vi "TIRF-Lock.vi"(8 "error in (no error)":errorcluster, 11 "Config":T1 {"Hardware Configuration"."Lasers Configuration"."SettingValues"."785 Power" format="%.1f"; "Hardware Configuration"."Lasers Configuration"."SettingValues"."647 Power" format="%.1f"; "Hardware Configuration"."Lasers Configuration"."SettingValues"."561 Power" format="%.1f"; "Hardware Configuration"."Lasers Configuration"."SettingValues"."532 Power" format="%.1f"; "Hardware Configuration"."Lasers Configuration"."SettingValues"."488 Power" format="%.1f"; "Hardware Configuration"."Lasers Configuration"."SettingValues"."405 Power" format="%.1f"}) -> (0 "error Out":errorcluster, 3 "Config 2":T1 {"Hardware Configuration"."Lasers Configuration"."SettingValues"."785 Power" format="%.1f"; "Hardware Configuration"."Lasers Configuration"."SettingValues"."647 Power" format="%.1f"; "Hardware Configuration"."Lasers Configuration"."SettingValues"."561 Power" format="%.1f"; "Hardware Configuration"."Lasers Configuration"."SettingValues"."532 Power" format="%.1f"; "Hardware Configuration"."Lasers Configuration"."SettingValues"."488 Power" format="%.1f"; "Hardware Configuration"."Lasers Configuration"."SettingValues"."405 Power" format="%.1f"})   [LabVIEW 2019]
uses:
  Settings/Settings.ctl
  HardwareAdapter/Support/Hardware Configuration.ctl
  HardwareAdapter/Support/Camera Configuration.ctl
  D:/SDK/PMQI-LabViewSamples/Examples/Dependencies/PVCamNET.dll
  <vilib>/vision/Image Controls.llb/IMAQ Image.ctl
  <vilib>/userdefined/High Color/IMAQdx.ctl
  E:/DevHardSoftware/MMicroscopy/HardwareAdapter/Lasers/Dependencies/Oxxius_Boxx.dll
  HardwareAdapter/Lasers/Dependencies/Oxxius_Boxx.dll
  Logging/Logging Configuration.ctl
  controls/UI Configuration.ctl
  controls/CallBack Refs.ctl
  Global.vi
  Logging/Logging.lvlib
  Settings/Settings.lvlib
panel:
  in  "Sum":dbl=0.01
  out "Lock Point Y":dbl step=0.01 format="%#.4g"
  out "Lock Point X":dbl step=0.01 format="%#.4g"
  out "cal":dbl format="%#.4g"
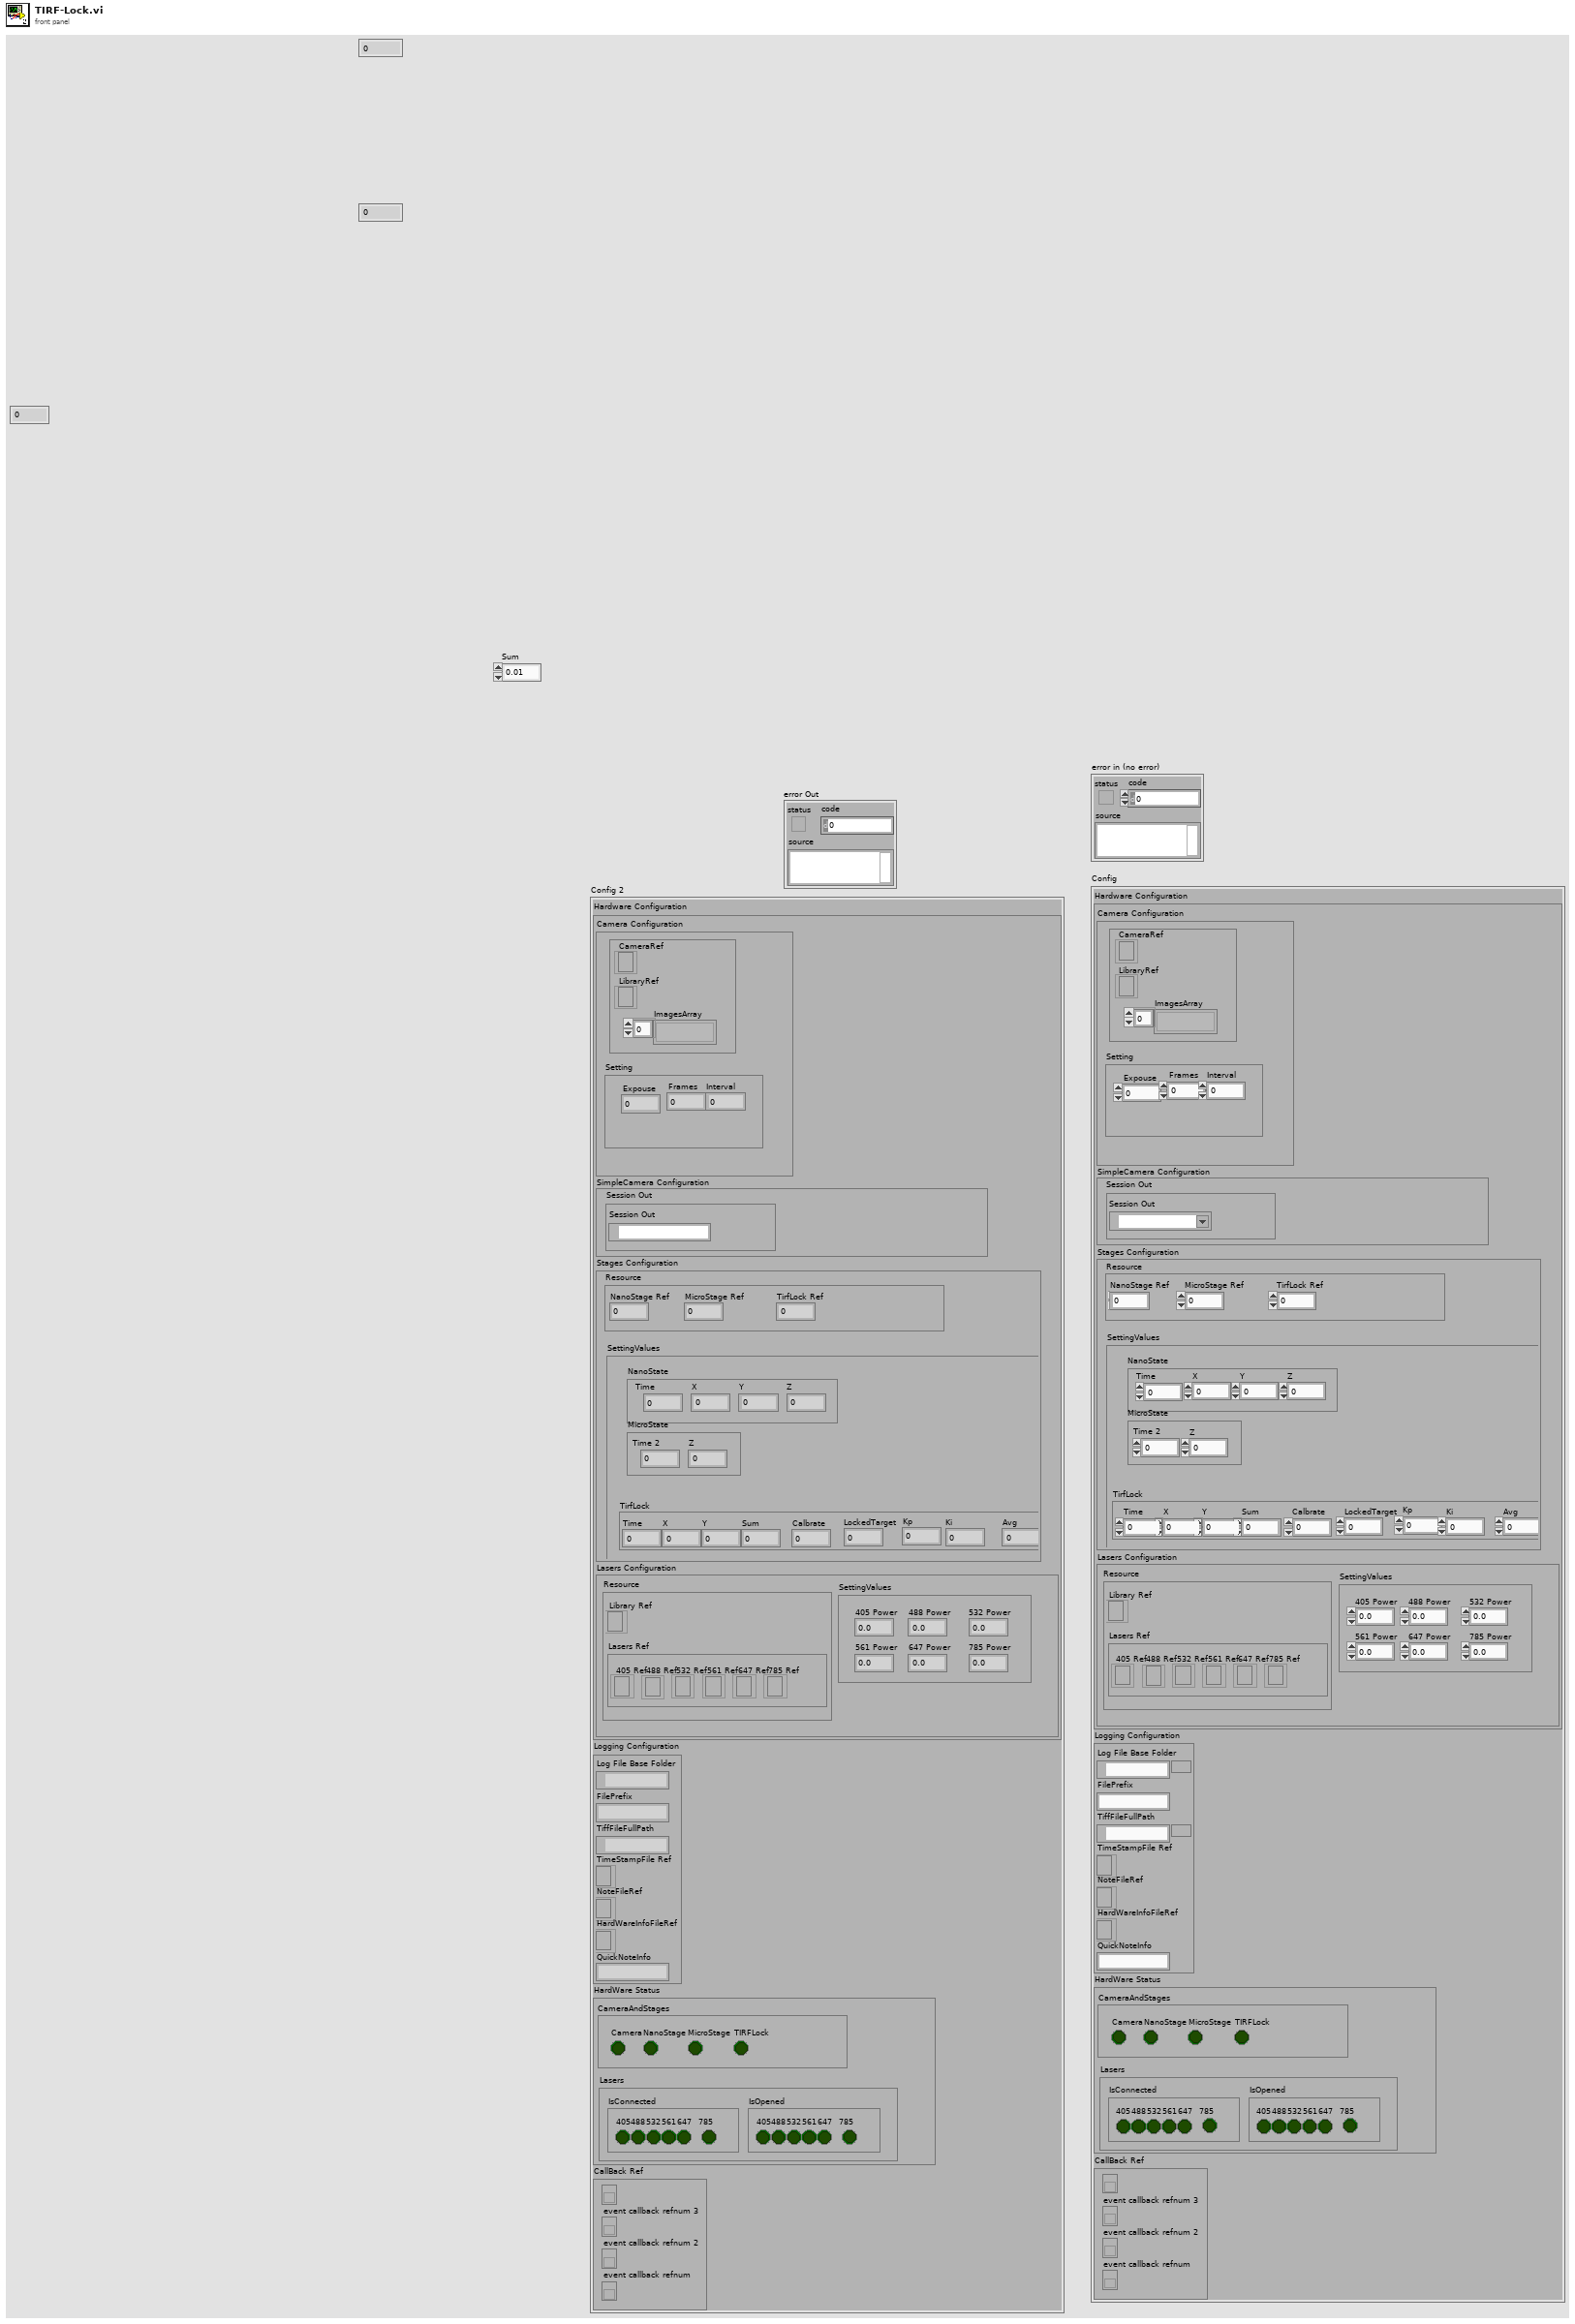
[diagram p1: front panel]
types:
  T1 = typedef "Settings.lvlib/Settings.ctl" = cluster{"Hardware Configuration":T2, "Logging Configuration":T6, "HardWare Status":cluster{"CameraAndStages":T7, "Lasers":cluster{"IsConnected":cluster{"405":bool, "488":bool, "532":bool, "561":bool, "647":bool, "785":bool}, "IsOpened":cluster{"405":bool, "488":bool, "532":bool, "561":bool, "647":bool, "785":bool}}}, "CallBack Ref":T8}
  T2 = typedef "Hardware Configuration.ctl" = cluster{"Camera Configuration":T3, "SimpleCamera Configuration":cluster{"Resource":cluster{"Session Out":T5}}, "Stages Configuration":cluster{"Resource":cluster{"NanoStage Ref":i32, "MicroStage Ref":i32, "TirfLock Ref":i32}, "SettingValues":cluster{"NanoState":cluster{"Time":dbl, "X":dbl, "Y":dbl, "Z":dbl}, "MicroState":cluster{"Time 2":dbl, "Z":dbl}, "TirfLock":cluster{"Time":dbl, "X":dbl, "Y":dbl, "Sum":dbl, "Calbrate":dbl, "LockedTarget":dbl, "Kp":dbl, "Ki":dbl, "Avg":dbl}}}, "Lasers Configuration":cluster{"SettingValues":cluster{"405 Power":sgl, "488 Power":sgl, "532 Power":sgl, "561 Power":sgl, "647 Power":sgl, "785 Power":sgl}, "Resource":cluster{"Library Ref":refnum<k24>, "Lasers Ref":cluster{"405 Ref":refnum<k24>, "488 Ref":refnum<k24>, "532 Ref":refnum<k24>, "561 Ref":refnum<k24>, "647 Ref":refnum<k24>, "785 Ref":refnum<k24>}}}}
  T3 = typedef "Camera Configuration.ctl" = cluster{"Setting":cluster{"Expouse":dbl, "Frames":dbl, "Interval":dbl}, "Resource":cluster{"CameraRef":refnum<k24>, "LibraryRef":refnum<k24>, "ImagesArray":T4[]}}
  T4 = typedef "IMAQ Image.ctl" = refnum<image>
  T5 = typedef "IMAQdx.ctl" = refnum<k21>
  T6 = typedef "Logging.lvlib/Logging Configuration.ctl" = cluster{"Log File Base Folder":path, "FilePrefix":string, "TiffFileFullPath":path, "TimeStampFile Ref":refnum<file>, "NoteFileRef":refnum<file>, "HardWareInfoFileRef":refnum<file>, "QuickNoteInfo":string}
  T7 = typedef "UI Configuration.ctl" = cluster{"Camera":bool, "NanoStage":bool, "MicroStage":bool, "TIRFLock":bool}
  T8 = typedef "CallBack Refs.ctl" = cluster{"event callback refnum":refnum<k27>, "event callback refnum 2":refnum<k27>, "event callback refnum 3":refnum<k27>, "event callback refnum 4":refnum<k27>}
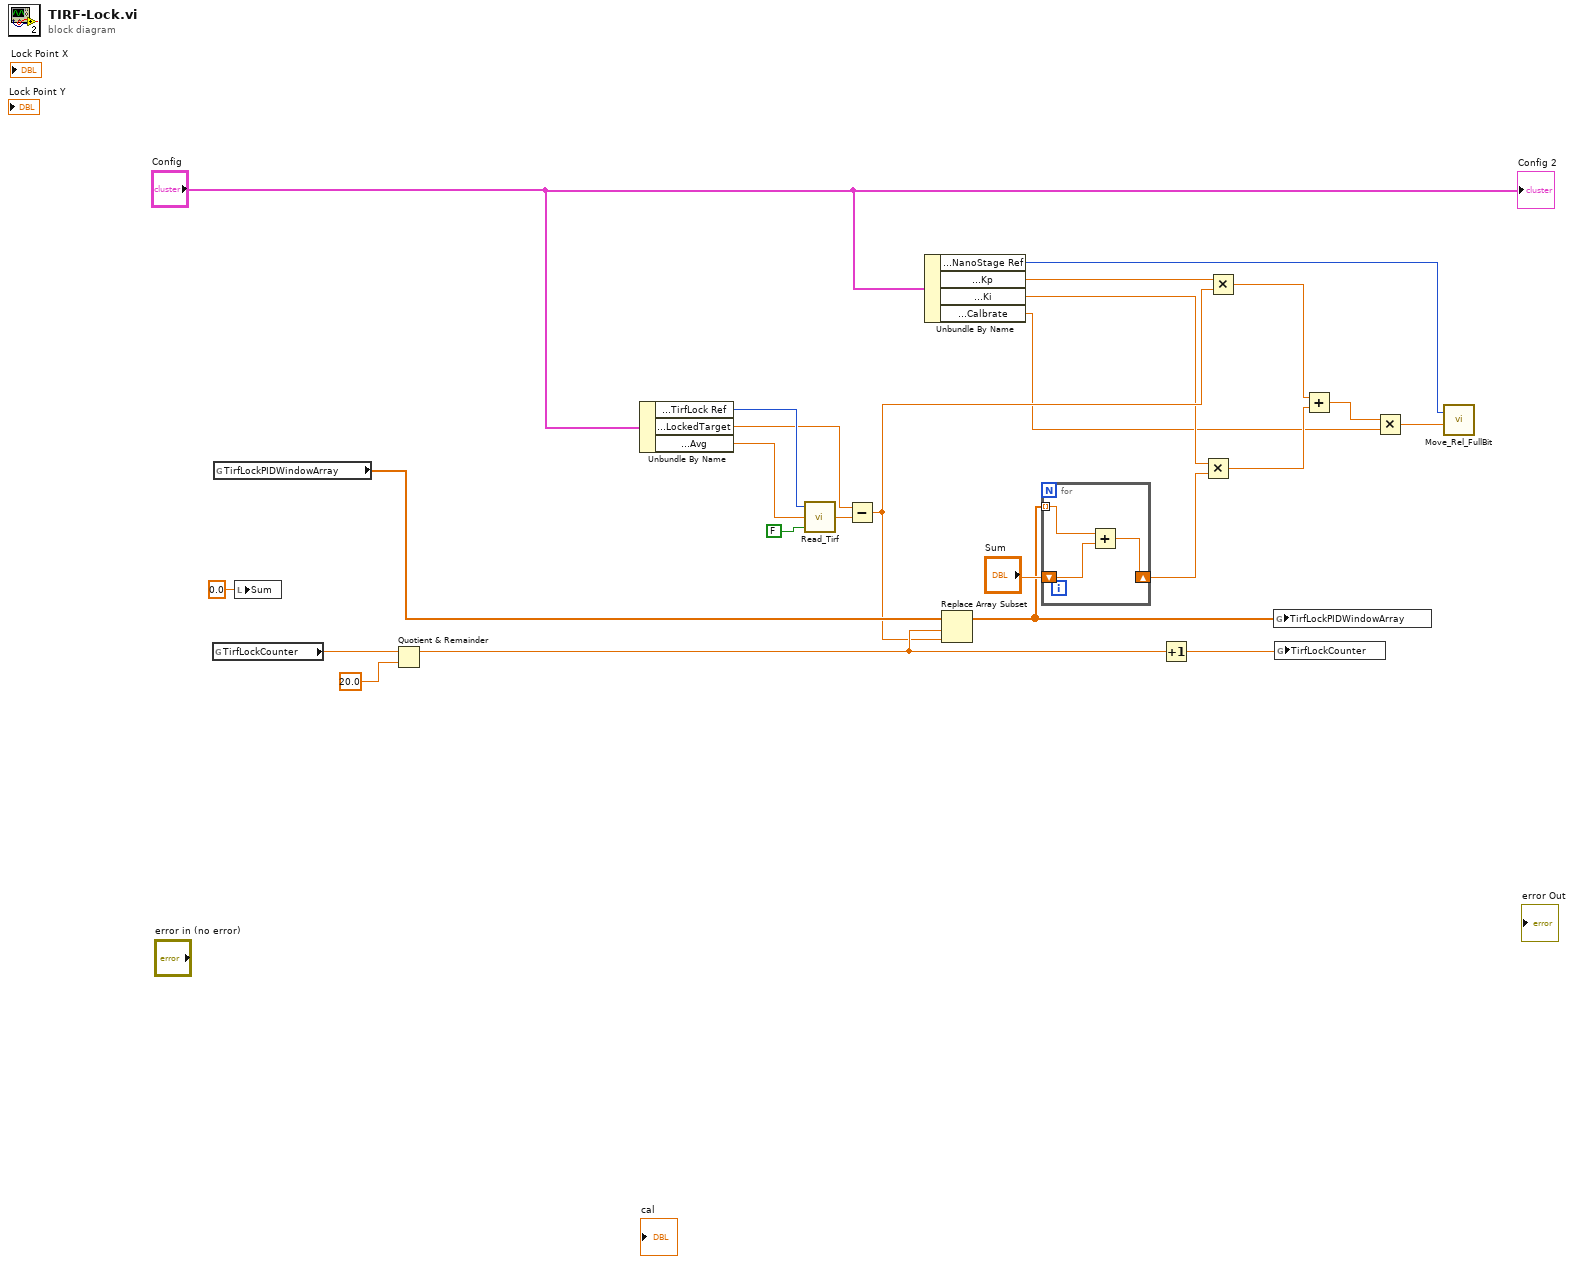
[diagram p0: block diagram]
diagram:
  n1 = global read "Global.vi" "TirfLockCounter"() -> (w16:dbl)
  n2 = global read "Global.vi" "TirfLockPIDWindowArray"() -> (w13:dbl[])
  n3 = local write "Sum"(0.0 ("Sum")) -> ()
  n4 = Quotient & Remainder(x=w16, y=20.0) -> (x-y*floor(x/y)=w12:dbl)  [unwired: 1 out]
  n5 = Unbundle By Name("Config") -> ("Hardware Configuration.Stages Configuration.Resource.TirfLock Ref"=w22:i32, "Hardware Configuration.Stages Configuration.SettingValues.TirfLock.LockedTarget"=w21:dbl, "Hardware Configuration.Stages Configuration.SettingValues.TirfLock.Avg"=w10:dbl)
  n6 = call "Read_Tirf.vi"("Display"=FALSE, "Averages"=w10, "Tirf-Handle"=w22) -> ("coerced(y)"=w23:dbl)  [unwired: 2 out]
  n7 = Subtract(x=w21, y=w23) -> (x-y=w6:dbl)
  n8 = Unbundle By Name("Config") -> ("Hardware Configuration.Stages Configuration.Resource.NanoStage Ref"=w1:i32, "Hardware Configuration.Stages Configuration.SettingValues.TirfLock.Kp"=w7:dbl, "Hardware Configuration.Stages Configuration.SettingValues.TirfLock.Ki"=w5:dbl, "Hardware Configuration.Stages Configuration.SettingValues.TirfLock.Calbrate"=w2:dbl)
  n9 = Replace Array Subset(array=w13, new element=w6, index=w12) -> (w11:dbl[])
  n10 = for {
    tunnel: w11 -> [w27] mode=indexing
    shift-right: [w25] -> w4
    shift-left: "Sum" -> [w26]
    n11 = Add(x=w27, y=w26) -> (x+y=w25:dbl)
  }
  n12 = Increment(x=w12) -> (x+1=w14:dbl)
  n13 = Multiply(x=w5, y=w4) -> (x*y=w19:dbl)
  n14 = Multiply(x=w7, y=w6) -> (x*y=w20:dbl)
  n15 = global write "Global.vi" "TirfLockPIDWindowArray"(w11) -> ()
  n16 = global write "Global.vi" "TirfLockCounter"(w14) -> ()
  n17 = Add(x=w20, y=w19) -> (x+y=w3:dbl)
  n18 = Multiply(x=w3, y=w2) -> (x*y=w24:dbl)
  n19 = call "Move_Rel_FullBit.vi"("relative Z"=w24, "handle"=w1) -> ()  [unwired: 2 in]
  "Config 2" <- "Config"
